vi "更新棋盘和棋子数据.vi"(0 "原始位置X":u8, 1 "到达的X":u8, 2 "游戏":T1, 3 "原始位置Y":u8, 4 "到达的Y":u8) -> (5 "游戏 2":T1)   [LabVIEW 2017]
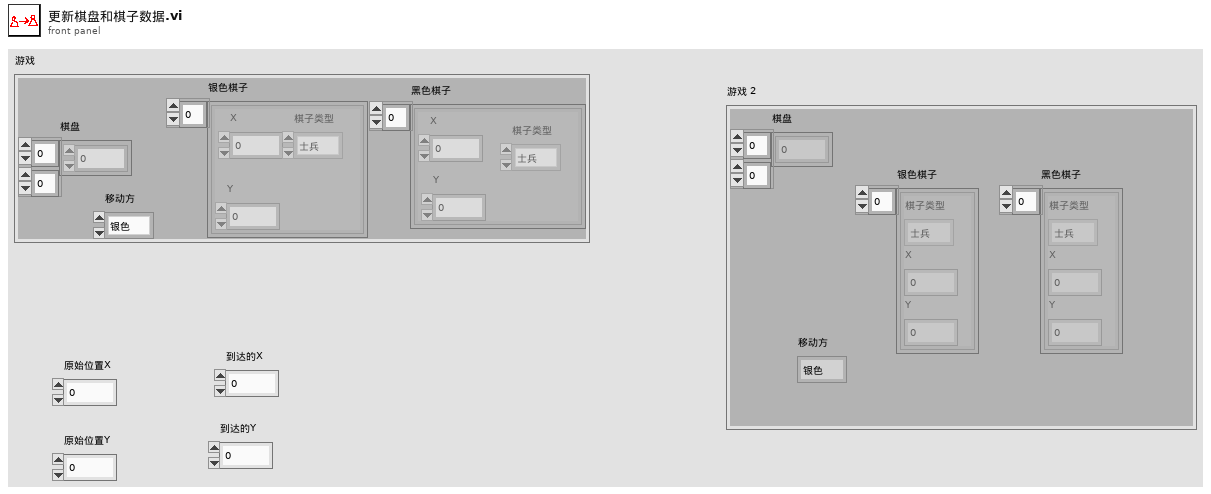
[diagram p1: front panel]
types:
  T1 = cluster{"棋盘":u16[][], "银色棋子":cluster{"棋子类型":enum16{"士兵", "骑士", "主教", "战车", "皇后", "国王", "空"}, "X":u8, "Y":u8}[], "黑色棋子":cluster{"棋子类型":enum16{"士兵", "骑士", "主教", "战车", "皇后", "国王", "空"}, "X":u8, "Y":u8}[], "移动方":enum16{"银色", "黑色"}}
  T2 = cluster{"棋子类型":enum16{"士兵", "骑士", "主教", "战车", "皇后", "国王", "空"}, "X":u8, "Y":u8}[]
  T3 = cluster{"棋子类型":enum16{"士兵", "骑士", "主教", "战车", "皇后", "国王", "空"}, "原始位置X":u8, "原始位置Y":u8}
  T4 = cluster{"棋子类型":enum16{"士兵", "骑士", "主教", "战车", "皇后", "国王", "空"}, "到达的X":u8, "到达的Y":u8}
  T5 = cluster{"棋盘":u16[][], "银色棋子":cluster{"棋子类型":enum16{"士兵", "骑士", "主教", "战车", "皇后", "国王", "空"}, "X":u8, "Y":u8}[], "黑色棋子":cluster{"棋子类型":enum16{"士兵", "骑士", "主教", "战车", "皇后", "国王", "空"}, "X":u8, "Y":u8}[], "y":enum16{"银色", "黑色"}}
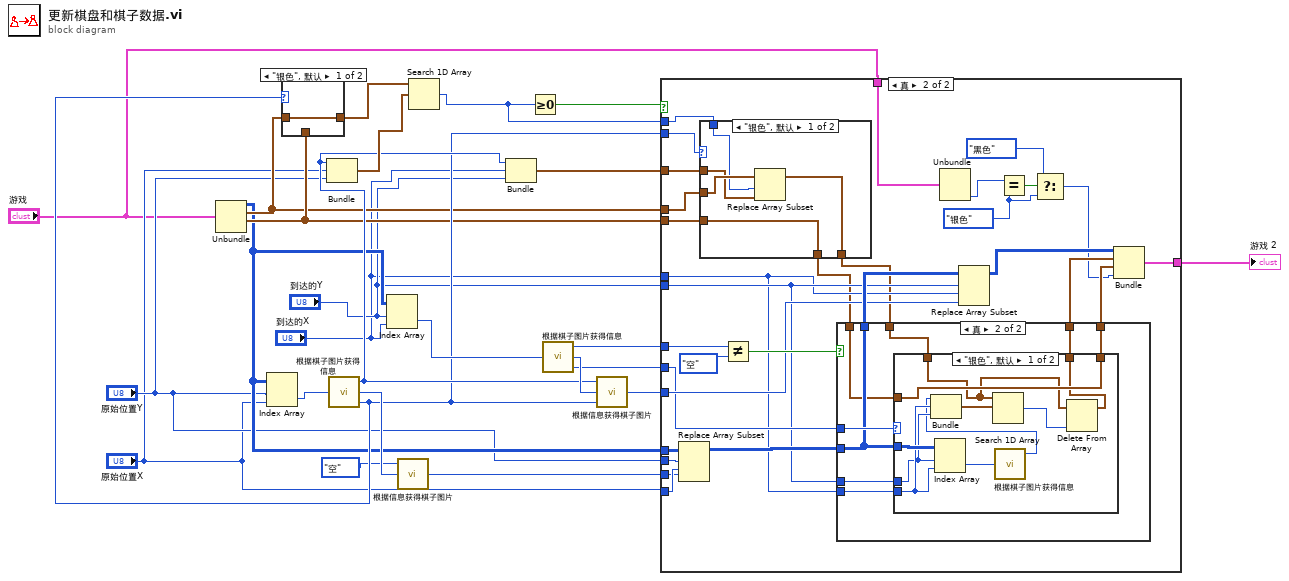
[diagram p0: block diagram]
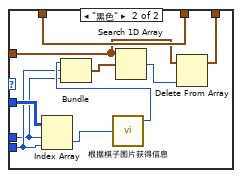
[diagram p4: hidden frame]
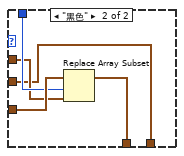
[diagram p5: hidden frame]
diagram:
  n1 = Unbundle("游戏") -> ("棋盘"=w12:u16[][], "银色棋子"=w13:T2, "黑色棋子"=w16:T2)  [unwired: 1 out]
  n2 = Index Array(array=w12, index (row)="原始位置Y", index (col)="原始位置X") -> (element=w25:u16)
  n3 = call "根据棋子图片获得信息.vi"("棋子"=w25) -> ("棋子类型"=w19:enum16{"士兵", "骑士", "主教", "战车", "皇后", "国王", "空"}, "背景颜色"=w24:enum16{"白色", "绿色"}, "棋子颜色"=w17:enum16{"银色", "黑色"})
  n4 = case shown="\"银色\", 默认" w17 {
    tunnel: [w26 w27] -> w21
    tunnel: w13 -> [w26 _]
    tunnel: w16 -> [_ w27]
    frame "银色", Default {
    }
    frame "黑色" {
    }
  }
  n5 = Bundle("棋子类型"=w19, "原始位置X"="原始位置X", "原始位置Y"="原始位置Y") -> (w20:T3)  [unwired: 1 in]
  n6 = Index Array(array=w12, index (row)="到达的Y", index (col)="到达的X") -> (element=w23:u16)
  n7 = call "根据信息获得棋子图片.vi"("背景颜色"=w24, "棋子类型"=enum16{"士兵", "骑士", "主教", "战车", "皇后", "国王", "空"}."空") -> ("棋子"=w9:u16)  [unwired: 1 in]
  n8 = Search 1D Array(1D array=w21, element=w20) -> (index of element=w15:i32)  [unwired: 1 in]
  n9 = Bundle("棋子类型"=w19, "到达的X"="到达的X", "到达的Y"="到达的Y") -> (w14:T4)  [unwired: 1 in]
  n10 = Greater Or Equal To 0?(x=w15) -> (x >= 0?=w18:bool)
  n11 = call "根据棋子图片获得信息.vi"("棋子"=w23) -> ("棋子类型"=w8:enum16{"士兵", "骑士", "主教", "战车", "皇后", "国王", "空"}, "背景颜色"=w22:enum16{"白色", "绿色"}, "棋子颜色"=w4:enum16{"银色", "黑色"})
  n12 = call "根据信息获得棋子图片.vi"("棋子颜色"=w17, "背景颜色"=w22, "棋子类型"=w19) -> ("棋子"=w5:u16)
  n13 = case shown="真" w18 {
    tunnel: w17 -> [_ w58]
    tunnel: w16 -> [_ w57]
    tunnel: w15 -> [_ w56]
    tunnel: w14 -> [_ w55]
    tunnel: w13 -> [_ w54]
    tunnel: "游戏" -> [w28 w53]
    tunnel: w12 -> [_ w50]
    tunnel: "原始位置Y" -> [_ w49]
    tunnel: "原始位置X" -> [_ w48]
    tunnel: w9 -> [_ w47]
    tunnel: w8 -> [_ w46]
    tunnel: "到达的Y" -> [_ w39]
    tunnel: "到达的X" -> [_ w38]
    tunnel: w5 -> [_ w41]
    tunnel: w4 -> [_ w40]
    tunnel: [w28 w31] -> w1
    frame False {
    }
    frame True {
      w30 = enum16{"银色", "黑色"}."银色" ("y")
      n14 = Replace Array Subset(array=w50, new element=w47, index (row)=w49, index (col)=w48) -> (w43:u16[][])
      n15 = case shown="\"银色\", 默认" w58 {
        tunnel: w57 -> [w90 w99]
        tunnel: w56 -> [w93 w98]
        tunnel: w55 -> [w92 w97]
        tunnel: [w90 w96] -> w37
        tunnel: [w91 w95] -> w36
        tunnel: w54 -> [w94 w95]
        frame "银色", Default {
          n16 = Replace Array Subset(array=w94, new element=w92, index=w93) -> (w91:T2)
        }
        frame "黑色" {
          n17 = Replace Array Subset(array=w99, new element=w97, index=w98) -> (w96:T2)
        }
      }
      n18 = Not Equal?(x=w46, y=enum16{"士兵", "骑士", "主教", "战车", "皇后", "国王", "空"}."空") -> (x != y?=w44:bool)
      n19 = case shown="真" w44 {
        tunnel: w43 -> [w61 w68]
        tunnel: [w61 w68] -> w42
        tunnel: w40 -> [_ w69]
        tunnel: w39 -> [_ w67]
        tunnel: w38 -> [_ w66]
        tunnel: w37 -> [w59 w65]
        tunnel: w36 -> [w60 w64]
        tunnel: [w60 w63] -> w35
        tunnel: [w59 w62] -> w34
        frame False {
        }
        frame True {
          n20 = case shown="\"银色\", 默认" w69 {
            tunnel: w68 -> [w79 w89]
            tunnel: w67 -> [w77 w85]
            tunnel: w66 -> [w78 w86]
            tunnel: w65 -> [w74 w81]
            tunnel: w64 -> [w71 w84]
            tunnel: [w70 w84] -> w63
            tunnel: [w74 w80] -> w62
            frame "银色", Default {
              n21 = Index Array(array=w79, index (row)=w77, index (col)=w78) -> (element=w76:u16)
              n22 = call "根据棋子图片获得信息.vi"("棋子"=w76) -> ("棋子类型"=w75:enum16{"士兵", "骑士", "主教", "战车", "皇后", "国王", "空"})  [unwired: 2 out]
              n23 = Bundle("棋子类型"=w75, "到达的X"=w78, "到达的Y"=w77) -> (w73:T4)  [unwired: 1 in]
              n24 = Search 1D Array(1D array=w71, element=w73) -> (index of element=w72:i32)  [unwired: 1 in]
              n25 = Delete From Array(array=w71, index=w72) -> (array with subset deleted=w70:T2)  [unwired: 1 in, 1 out]
            }
            frame "黑色" {
              n26 = Index Array(array=w89, index (row)=w85, index (col)=w86) -> (element=w88:u16)
              n27 = call "根据棋子图片获得信息.vi"("棋子"=w88) -> ("棋子类型"=w87:enum16{"士兵", "骑士", "主教", "战车", "皇后", "国王", "空"})  [unwired: 2 out]
              n28 = Bundle("棋子类型"=w87, "到达的X"=w86, "到达的Y"=w85) -> (w83:T4)  [unwired: 1 in]
              n29 = Search 1D Array(1D array=w81, element=w83) -> (index of element=w82:i32)  [unwired: 1 in]
              n30 = Delete From Array(array=w81, index=w82) -> (array with subset deleted=w80:T2)  [unwired: 1 in, 1 out]
            }
          }
        }
      }
      n31 = Unbundle(w53) -> ("移动方"=w52:enum16{"银色", "黑色"})  [unwired: 3 out]
      n32 = Replace Array Subset(array=w42, new element=w41, index (row)=w39, index (col)=w38) -> (w33:u16[][])
      n33 = Equal?(x=w52, y=w30) -> (x = y?=w51:bool)
      n34 = Select(t=enum16{"银色", "黑色"}."黑色", s=w51, f=w30) -> (s? t:f=w32:enum16{"银色", "黑色"})
      n35 = Bundle("棋盘"=w33, "银色棋子"=w35, "黑色棋子"=w34, "y"=w32) -> (w31:T5)  [unwired: 1 in]
    }
  }
  "游戏 2" <- w1
